vi "MainStateMachine.vi"() -> ()   [LabVIEW 2014]
uses:
  Controls/StateControl.ctl
  <vilib>/Instr/_visa.llb/VISA Configure Serial Port (Instr).vi
  <vilib>/MakerHub/LINX/Public/Utilities/Open Local.vi
  <vilib>/MakerHub/LINX/LMH-LINX.lvlib
panel:
  out "Reset":u8[](array[numeric]) format="%x"
  out "Reset Response":string
  out "Get Health":u8[](array[numeric]) format="%x"
  out "Health Response":string
  out "Payload":u8[](array[numeric])
  out "Header":u8[](array[numeric])
  out "Size":u32
  in  "RESET":bool
  in  "GET HEALTH":bool
  in  "EXIT":bool
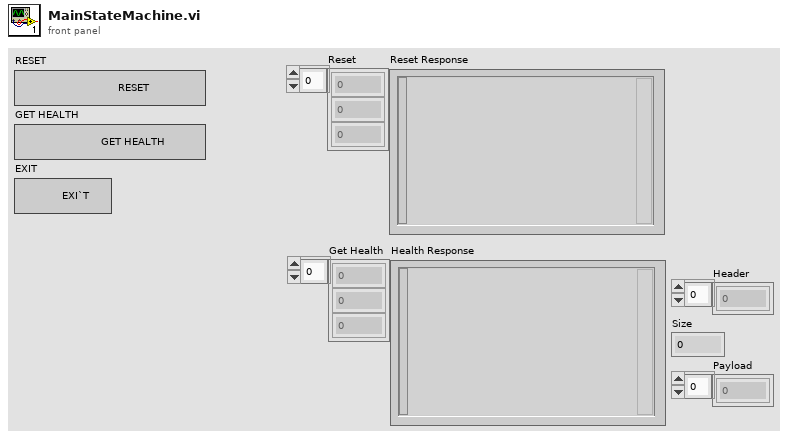
[diagram p1: front panel]
types:
  T1 = typedef "StateControl.ctl" = enum16{"WAIT FOR EVENT", "GET HEALTH", "SCAN", "RESET", "EXIT"}
  T2 = typedef "LMH-LINX.lvlib/LINX Ref.ctl" = cluster{"IO":T3, "Interface":T4, "LINX Device Config":T5}
  T3 = typedef "LMH-LINX.lvlib/Platform.ctl" = enum16{"Remote", "Local"}
  T4 = typedef "LMH-LINX.lvlib/Interface.ctl" = enum16{"Serial", "TCP"}
  T5 = typedef "LMH-LINX.lvlib/Device.lvlib/LINX Device Config.ctl" = cluster{"Interface":T4, "COM Port":refnum<visa-resource-name>, "TCP Configuration":T6, "Device Family":u8, "Device ID":u8, "Device Name":string, "TCP Ref":refnum<k5>, "Channels":T7}
  T6 = typedef "LMH-LINX.lvlib/Device.lvlib/TCP Config.ctl" = cluster{"IP Address":string, "Port":u16}
  T7 = typedef "LMH-LINX.lvlib/Channels.ctl" = cluster{"DI":u8[], "DO":u8[], "AI":u8[], "AO":u8[], "PWM":u8[], "QE":u8[], "UART":u8[], "I2C 2":u8[], "SPI":u8[], "CAN":u8[], "Servo":u8[], "AI Ref (V)":dbl, "AI Resolution (Bits)":u8, "AO Ref (V)":dbl, "AO Resolution (Bits)":u8}
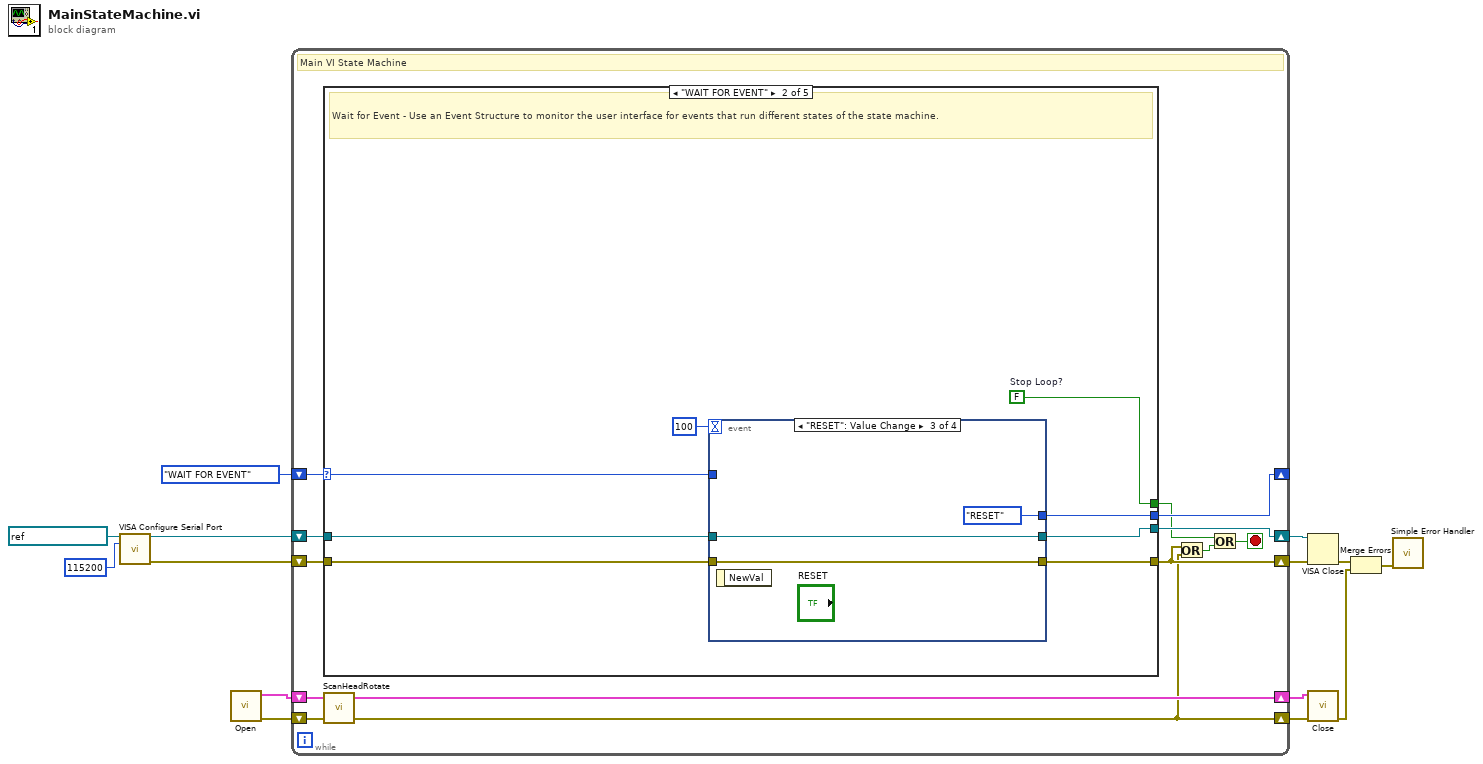
[diagram p0: block diagram]
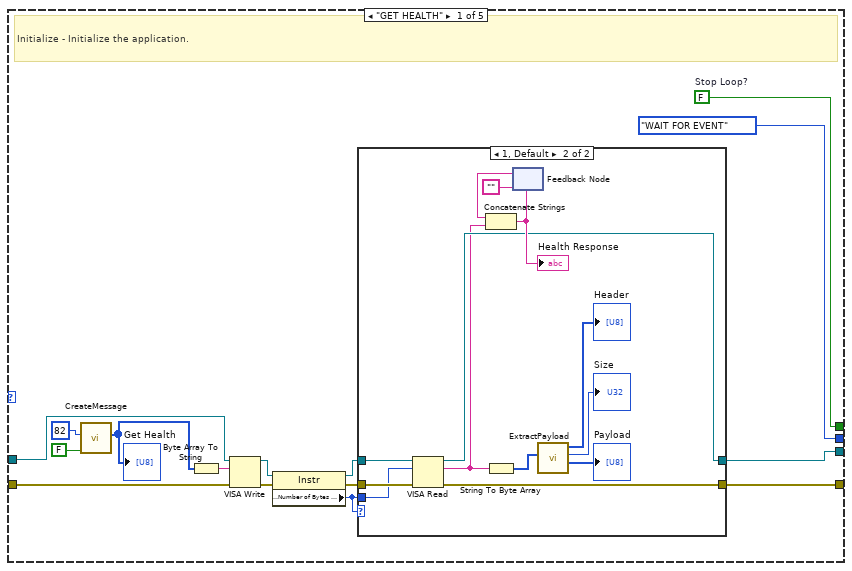
[diagram p2: hidden frame]
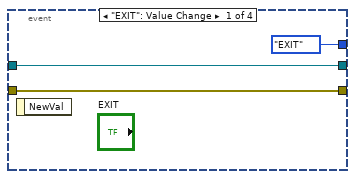
[diagram p4: hidden frame]
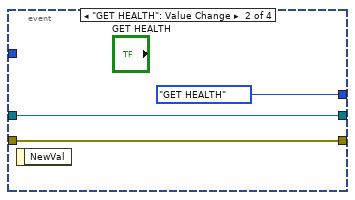
[diagram p5: hidden frame]
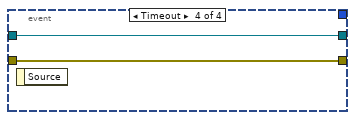
[diagram p6: hidden frame]
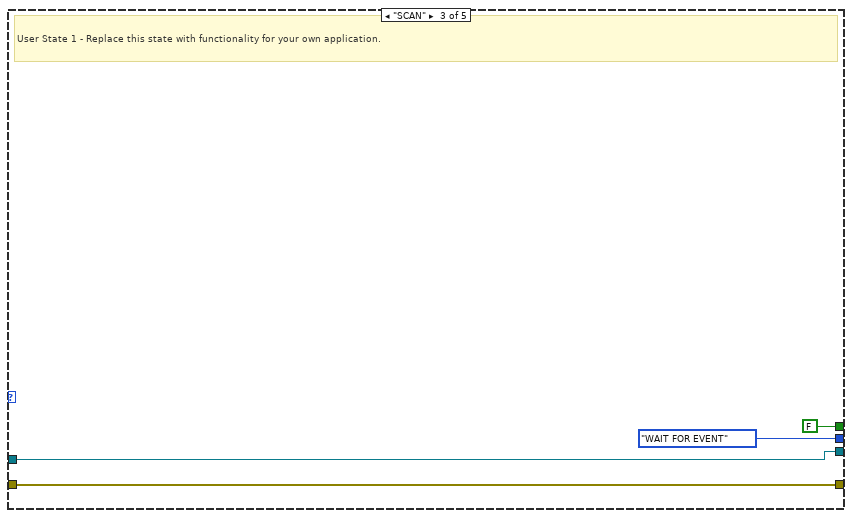
[diagram p7: hidden frame]
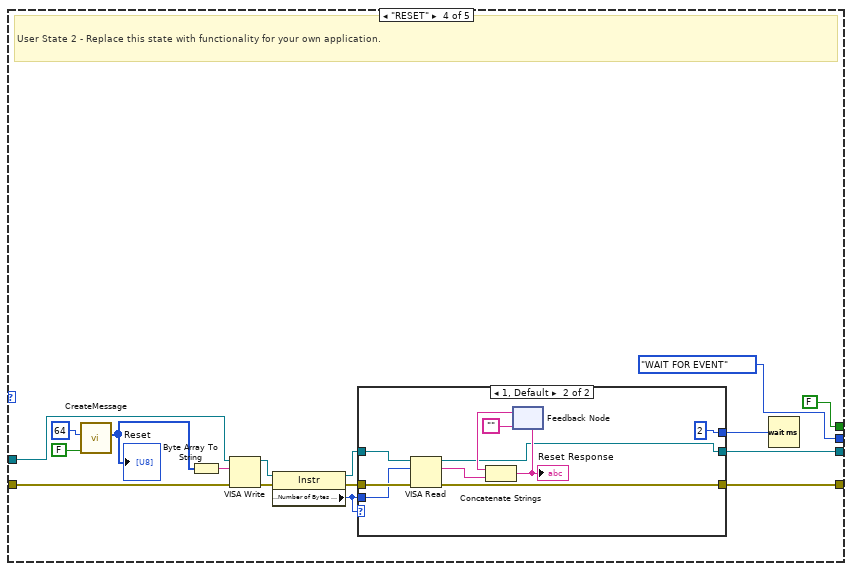
[diagram p8: hidden frame]
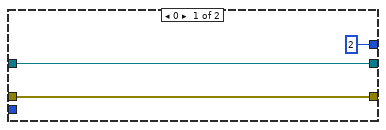
[diagram p9: hidden frame]
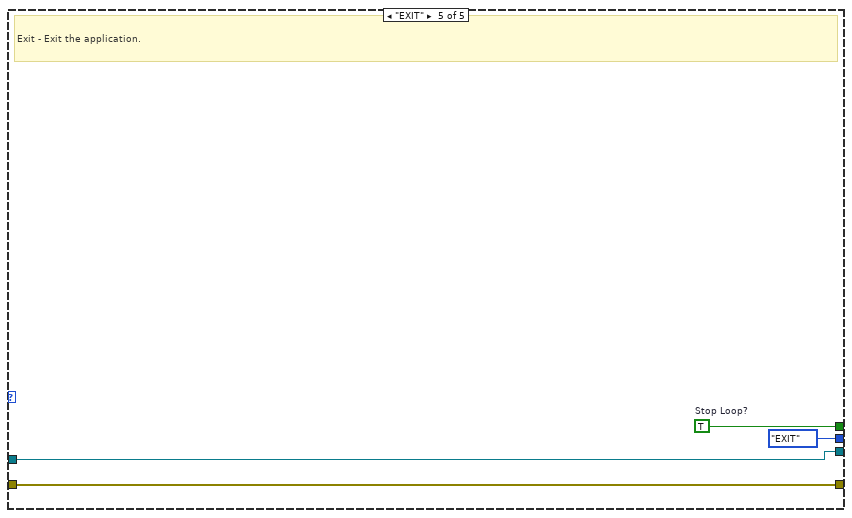
[diagram p10: hidden frame]
diagram:
  n1 = call-poly "VISA Configure Serial Port"("VISA resource name"=refnum<visa-resource-name> "ASRL3::INSTR", "baud rate (9600)"=u32 115200) -> ("VISA resource name out"=w7:refnum<visa-resource-name>, "error out"=w8:errorcluster)  [unwired: 8 in, 4 out]
  n2 = call-poly <vilib>:"Open.vi"() -> ("Error Out"=w5:errorcluster, "LINX Resource"=w4:T2)  [unwired: 9 in, 1 out]
  n3 = while {
    shift-right: [w17] -> w11
    shift-left: w8 -> [w27]
    shift-right: [w25] -> _
    shift-left: StateControl."WAIT FOR EVENT" -> [w26]
    shift-right: [w23] -> w6
    shift-left: w7 -> [w24]
    shift-right: [w20] -> w2
    shift-left: w4 -> [w21]
    shift-right: [w16] -> w1
    shift-left: w5 -> [w22]
    stop <- w19 stop-if-true
    # "Main VI State Machine"
    n4 = case shown="\"WAIT FOR EVENT\"" w26 {
      selector: w26 -> [_ w59 _ _ _]
      tunnel: [w42 w65 FALSE ("Stop Loop?") FALSE ("Stop Loop?") w113] -> w18
      tunnel: w27 -> [w30 w64 w79 w81 w112]
      tunnel: [w28 w63 w79 w84 w112] -> w17
      tunnel: [StateControl."WAIT FOR EVENT" w62 StateControl."WAIT FOR EVENT" StateControl."WAIT FOR EVENT" StateControl."EXIT"] -> w25
      tunnel: w24 -> [w31 w60 w77 w82 w110]
      tunnel: [w29 w61 w77 w83 w110] -> w23
      frame "GET HEALTH" {
        w42 = FALSE  # Stop Loop?
        # "Initialize - Initialize the application."
        n5 = call "CreateMessage.vi"("Calculate Checksum"=FALSE, "Command"=u8 82) -> ("Message"=w39:u8[])  [unwired: 9 in]
        "Get Health" <- w39
        n6 = Byte Array To String(unsigned byte array=w39) -> (string=w40:string)
        n7 = VISA Write(VISA resource name=w31, write buffer=w40, error in (no error)=w30) -> (VISA resource name out=w37:refnum<visa-resource-name>, error out=w36:errorcluster)  [unwired: 1 out]
        n8 = property class="Instr"(reference=w37, error in=w36) -> (reference out=w34:refnum<visa-resource-name>, error out=w33:errorcluster, "Serial Settings:Number of Bytes at Serial Port"=w32:u32)
        n9 = case shown="1, Default" w32 {
          tunnel: [w44 w54] -> w29
          tunnel: [w43 w53] -> w28
          tunnel: w34 -> [w44 w52]
          tunnel: w33 -> [w43 w51]
          tunnel: w32 -> [_ w50]
          frame 0 {
          }
          frame 1, Default {
            n10 = VISA Read(VISA resource name=w52, byte count=w50, error in (no error)=w51) -> (VISA resource name out=w54:refnum<visa-resource-name>, read buffer=w48:string, error out=w53:errorcluster)  [unwired: 1 out]
            n11 = String To Byte Array(string=w48) -> (unsigned byte array=w49:u8[])
            n12 = feedback #1("") -> (w57:string)
            n13 = Concatenate Strings(w57, w48) -> (w56:string)
            "Health Response" <- w56
            n14 = feedback-in #1(w56) -> ()
            n15 = call "ExtractPayload.vi"("Received Message"=w49) -> ("Payload"=→"Payload":u8[], "Size"=→"Size":u32, "Header"=→"Header":u8[])  [unwired: 7 in, 1 out]
          }
        }
      }
      frame "WAIT FOR EVENT" {
        w65 = FALSE  # Stop Loop?
        # "Wait for Event - Use an Event Structure to monitor the user interface for events that run different states of the state machine."
        n16 = event shown="[2] \"RESET\": Value Change" {
          selector: _ -> [_ _ _ _]
          dyn-events: _ -> [_ _ _ _]
          timeout: 100 -> [_ _ _ _]
          tunnel: w64 -> [w68 w71 w74 w76]
          tunnel: [w68 w71 w74 w76] -> w63
          tunnel: [StateControl."EXIT" StateControl."GET HEALTH" StateControl."RESET" _] -> w62
          tunnel: [w66 w69 w72 w75] -> w61
          tunnel: w60 -> [w66 w69 w72 w75]
          tunnel: w59 -> [_ _ _ _]
          event "EXIT": Value Change {
            n17 = event-data() -> ()  [unwired: 1 in, 1 out]
          }
          event "GET HEALTH": Value Change {
            n18 = event-data() -> ()  [unwired: 1 in, 1 out]
          }
          event "RESET": Value Change {
            n19 = event-data() -> ()  [unwired: 1 in, 1 out]
          }
          event Timeout {
            n20 = event-data() -> ()  [unwired: 1 in, 1 out]
          }
        }
      }
      frame "SCAN" {
        # "User State 1 - Replace this state with functionality for your own application."
      }
      frame "RESET" {
        # "User State 2 - Replace this state with functionality for your own application."
        n21 = call "CreateMessage.vi"("Calculate Checksum"=FALSE, "Command"=u8 64) -> ("Message"=w93:u8[])  [unwired: 9 in]
        "Reset" <- w93
        n22 = Byte Array To String(unsigned byte array=w93) -> (string=w94:string)
        n23 = VISA Write(VISA resource name=w82, write buffer=w94, error in (no error)=w81) -> (VISA resource name out=w89:refnum<visa-resource-name>, error out=w88:errorcluster)  [unwired: 1 out]
        n24 = property class="Instr"(reference=w89, error in=w88) -> (reference out=w91:refnum<visa-resource-name>, error out=w90:errorcluster, "Serial Settings:Number of Bytes at Serial Port"=w87:u32)
        n25 = case shown="1, Default" w87 {
          tunnel: [w99 w105] -> w83
          tunnel: [w98 w104] -> w84
          tunnel: w91 -> [w99 w103]
          tunnel: w90 -> [w98 w102]
          tunnel: w87 -> [_ w101]
          tunnel: [u32 2 ("milliseconds to wait") u32 2 ("milliseconds to wait")] -> w85
          frame 0 {
          }
          frame 1, Default {
            n26 = VISA Read(VISA resource name=w103, byte count=w101, error in (no error)=w102) -> (VISA resource name out=w105:refnum<visa-resource-name>, read buffer=w109:string, error out=w104:errorcluster)  [unwired: 1 out]
            n27 = feedback #2("") -> (w108:string)
            n28 = Concatenate Strings(w108, w109) -> (w107:string)
            "Reset Response" <- w107
            n29 = feedback-in #2(w107) -> ()
          }
        }
        n30 = Wait (ms)(milliseconds to wait=w85) -> ()  [unwired: 1 out]
      }
      frame "EXIT" {
        w113 = TRUE  # Stop Loop?
        # "Exit - Exit the application."
      }
    }
    n31 = call "ScanHeadRotate.vi"("Error In"=w22, "LINX Resource In"=w21) -> ("Error Out"=w16:errorcluster, "LINX Resource Out"=w20:T2)  [unwired: 2 in]
    n32 = Or(x=w17, y=w16) -> (x .or. y?=w15:bool)
    n33 = Or(x=w18, y=w15) -> (x .or. y?=w19:bool)
  }
  n34 = VISA Close(VISA resource name=w6, error in (no error)=w11) -> (error out=w10:errorcluster)
  n35 = call <vilib>:"Close.vi"("Error In"=w1, "LINX Resource"=w2) -> ("Error Out"=w3:errorcluster)  [unwired: 9 in]
  n36 = Merge Errors(w10, w3) -> (w9:errorcluster)
  n37 = call <vilib>:"Simple Error Handler.vi"("error in (no error)"=w9) -> ()  [unwired: 4 in, 5 out]
